vi "Slower PID.vi"(0 "process variable":i16, 1 "reset?":bool, 7 "setpoint":i16, 12 "PID gains (x 2^8)":T1={"proportional gain (Kc)"=1, "integral gain (Kc*Ts/Ti)"=0, "derivative gain (Kc*Td/Ts)"=0}, 13 "output range":cluster{"output high":i16, "output low":i16}={"output high"=2048, "output low"=0}) -> (4 "output":i16)   [LabVIEW 2014]
doc: "On an FPGA target, implements an integer PID algorithm for PID applications with high-speed control and/or high channel count that require an efficient algorithm. You can use this Express VI with single-channel or multi-channel configurations. The PID algorithm features control action range and uses the integrator anti-windup calculation to limit the effect of the integral action during transients. The PID algorithm also features bumpless controller output for PID gain changes.\n--------------------\n\nThis Express VI is configured as follows:\n\nNumber of channels = 1\nProportional gain (Kc) = 1\nIntegral time (Ti) = 10mmin\nDerivative time (Td) = 0min\nSampling time (Ts) = 20us\nProportional gain (scaled) (Kc * 2^8) = 256\nIntegral gain (scaled) ([Kc*Ts]/[Ti*60] * 2^8) = 0\nDerivative gain (scaled) ([Kc*Td*60]/[Ts] * 2^8) = 0\nOutput range high = 2048\nOutput range low = 0\nInitial setpoint = 0"
uses:
  <vilib>/Platform/TimedLoop/XDataNode/timing_clust.ctl
  <vilib>/Platform/TimedLoop/XDataNode/nitl_modes.ctl
  <vilib>/Platform/TimedLoop/XDataNode/wakeup.ctl
  <vilib>/rvi/Emulation/niFpgaSctlEmulationGetInTimedLoop.vi
  <vilib>/rvi/Emulation/niFpgaEmulationReportErrorSimple.vi
  <vilib>/rvi/Emulation/niFpgaGetClockAttributes.vi
  <vilib>/rvi/Emulation/niFpgaCriticalErrorInLSC.vi
  <vilib>/Platform/TimedLoop/XDataNode/XDataNode.xnode
  <vilib>/Platform/TimedLoop/XDataNode/XDNodeRunTimeDep.lvlib
  <vilib>/addons/control/pid/NI_PID_FPGA.lvlib
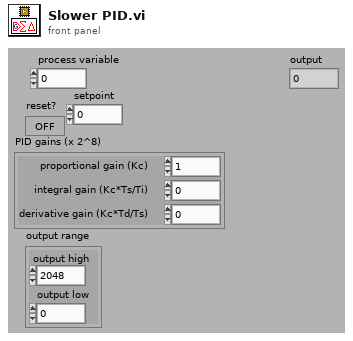
[diagram p1: front panel]
types:
  T1 = cluster{"proportional gain (Kc)":i16, "integral gain (Kc*Ts/Ti)":i16, "derivative gain (Kc*Td/Ts)":i16}
  T2 = typedef "XDNodeRunTimeDep.lvlib/timing_clust.ctl" = cluster{"Expected End [f-1]":u64, "Actual End [f-1]":u64, "Finished Late? [f-1]":bool, "Expected End [i-1]":u64, "Actual End [i-1]":u64, "Finished Late? [i-1]":bool, "Expected Start [i]":u64, "Actual Start [i]":u64, "Expected Start [f]":u64, "Actual Start [f]":u64, "Source Name":string, "Structure Name":string, "Period":i64, "Deadline":i64, "Offset":i64, "Start":i64, "Priority":i32, "Timeout":i32, "Mode":T3, "Wakeup Reason":T4, "Error":errorcluster, "Source Type":string, "Secondary Source Type":string, "Global End Time":u64, "Global Start Time":u64, "Frame Duration":u64, "Iteration Duration":u64, "Assigned CPU":i32, "I/O Scan Engine Mode":u32}
  T3 = typedef "XDNodeRunTimeDep.lvlib/nitl_modes.ctl" = enum32{"No Change", "Process missed periods, maintain original phase", "Discard missed periods, maintain original phase", "Process missed periods, ignore original phase", "Discard missed periods, ignore original phase"}
  T4 = typedef "XDNodeRunTimeDep.lvlib/wakeup.ctl" = enum32{"Normal", "Aborted", "Asynchronous wakeup", "Timing source error", "Timed loop error", "Timeout"}
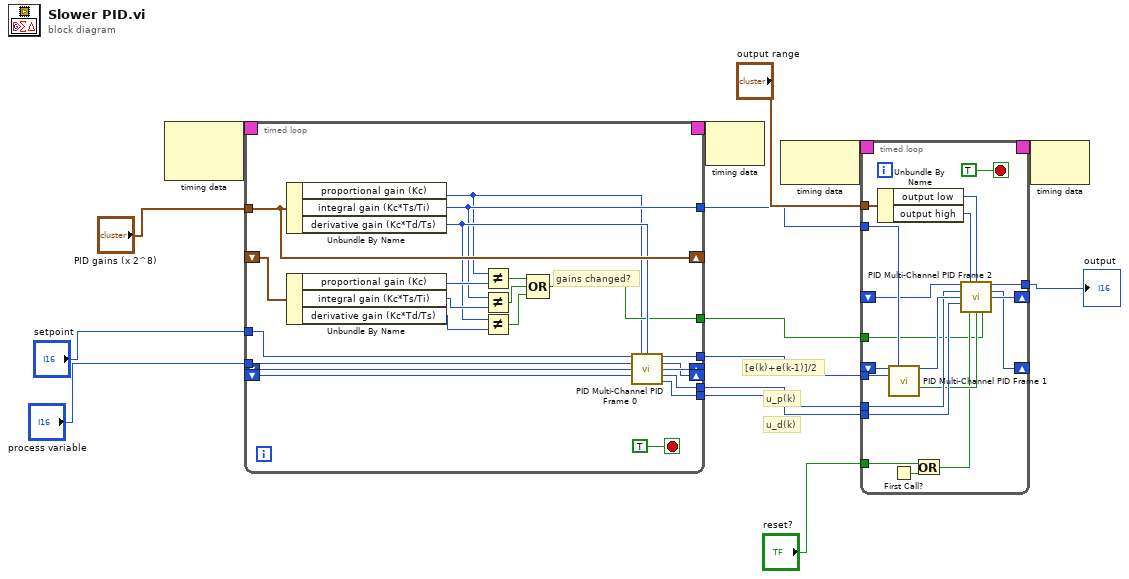
[diagram p0: block diagram]
diagram:
  # "u_d(k)"
  # "u_p(k)"
  # "[e(k)+e(k-1)]/2"
  n1 = node-c288() -> (w9:T2)  [unwired: 2 in]
  n2 = timed-loop {
    shift-right: [w36] -> _
    shift-left: _ -> [w35]
    timing: w9 -> [_]
    timing-out: [_] -> w8
    tunnel: "setpoint" -> [w27]
    tunnel: "process variable" -> [w26]
    tunnel: "PID gains (x 2^8)" -> [w36]
    shift-right: [w25] -> _
    shift-left: _ -> [w24]
    shift-right: [w22] -> _
    shift-left: _ -> [w23]
    tunnel: [w21] -> w3
    tunnel: [w20] -> w4
    tunnel: [w19] -> w5
    tunnel: [w18] -> w1
    tunnel: [w17] -> w2
    stop <- TRUE stop-if-true
    # "gains changed?"
    n3 = Unbundle By Name(w36) -> ("proportional gain (Kc)"=w16:i16, "integral gain (Kc*Ts/Ti)"=w18:i16, "derivative gain (Kc*Td/Ts)"=w28:i16)
    n4 = Unbundle By Name(w35) -> ("proportional gain (Kc)"=w34:i16, "integral gain (Kc*Ts/Ti)"=w32:i16, "derivative gain (Kc*Td/Ts)"=w30:i16)
    n5 = Not Equal?(x=w16, y=w34) -> (x != y?=w33:bool)
    n6 = Not Equal?(x=w18, y=w32) -> (x != y?=w31:bool)
    n7 = Not Equal?(x=w28, y=w30) -> (x != y?=w29:bool)
    n8 = Compound Arithmetic op=OR(w33, w31, w29) -> (w17:bool)
    n9 = call <vilib>:"PID Multi-Channel PID Frame 0.vi"("setpoint"=w27, "proportional gain (Kc) (k)"=w16, "derivative gain (Kc*Td/Ts) (k)"=w28, "PV(k)"=w26, "e(k-1)"=w24, "PV(k-1)"=w23) -> ("[e(k)+e(k-1)]/2"=w21:i16, "PV(k)"=w22:i16, "e(k)"=w25:i16, "u_p(k)"=w20:i32, "u_d(k)"=w19:i32)  [unwired: 5 out]
  }
  n10 = node-c288(w8) -> ()  [unwired: 1 out]
  n11 = node-c288() -> (w7:T2)  [unwired: 1 in]
  n12 = timed-loop {
    timing: w7 -> [_]
    timing-out: [_] -> w6
    tunnel: w1 -> [w57]
    tunnel: w4 -> [w55]
    tunnel: w5 -> [w54]
    tunnel: [w53] -> w13
    shift-right: [w52] -> _
    shift-left: _ -> [w48]
    tunnel: w2 -> [w40]
    shift-right: [w51] -> _
    shift-left: _ -> [w50]
    tunnel: w3 -> [w49]
    tunnel: "output range" -> [w46]
    tunnel: "reset?" -> [w42]
    stop <- TRUE stop-if-true
    n13 = Unbundle By Name(w46) -> ("output low"=w44:i16, "output high"=w45:i16)
    n14 = call <vilib>:"PID Multi-Channel PID Frame 1.vi"("ie(k-1)"=w50, "integral gain (Kc*Ts/Ti) (k)"=w57, "[e(k)+e(k-1)]/2"=w49) -> ("u_i(k)"=w56:i32, "integration off"=w47:bool)  [unwired: 11 out]
    n15 = First Call?() -> (First Call?: T/F=w43:bool)
    n16 = Or(x=w42, y=w43) -> (x .or. y?=w41:bool)
    n17 = call <vilib>:"PID Multi-Channel PID Frame 2.vi"("output(k-1)"=w48, "output range high"=w45, "output range low"=w44, "u_p(k)"=w55, "u_i(k)"=w56, "u_d(k)"=w54, "first call or initialize?"=w41, "integration off?"=w47, "gains changed?"=w40) -> ("output"=w53:i16, "integrated effort(k)"=w51:i32, "unscaled output(k)"=w52:i32)  [unwired: 4 out]
  }
  "output" <- w13
  n18 = node-c288(w6) -> ()  [unwired: 1 out]
